vi "WriteResults - Rx.vi"(8 "error in (no error)":errorcluster, 9 "PSR":dbl, 11 "refnum out":refnum<file>) -> (0 "error out":errorcluster, 3 "refnum out 2":refnum<file>)   [LabVIEW 2012]
panel:
  out "concatenated string":string
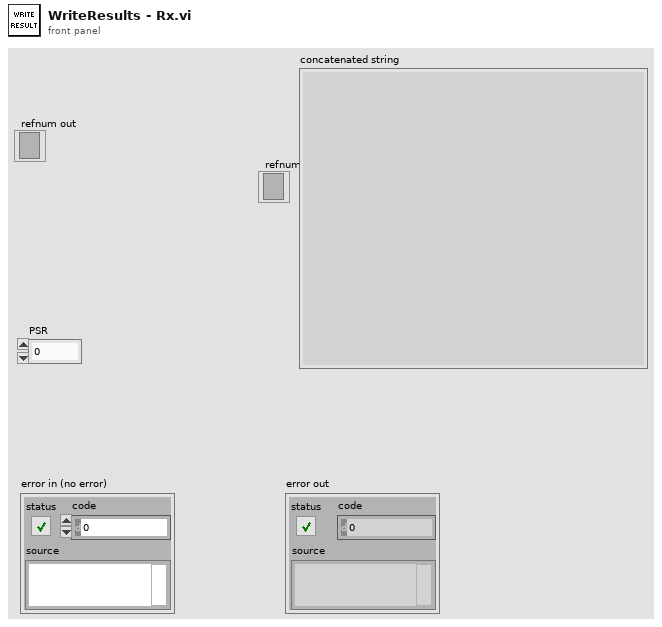
[diagram p1: front panel]
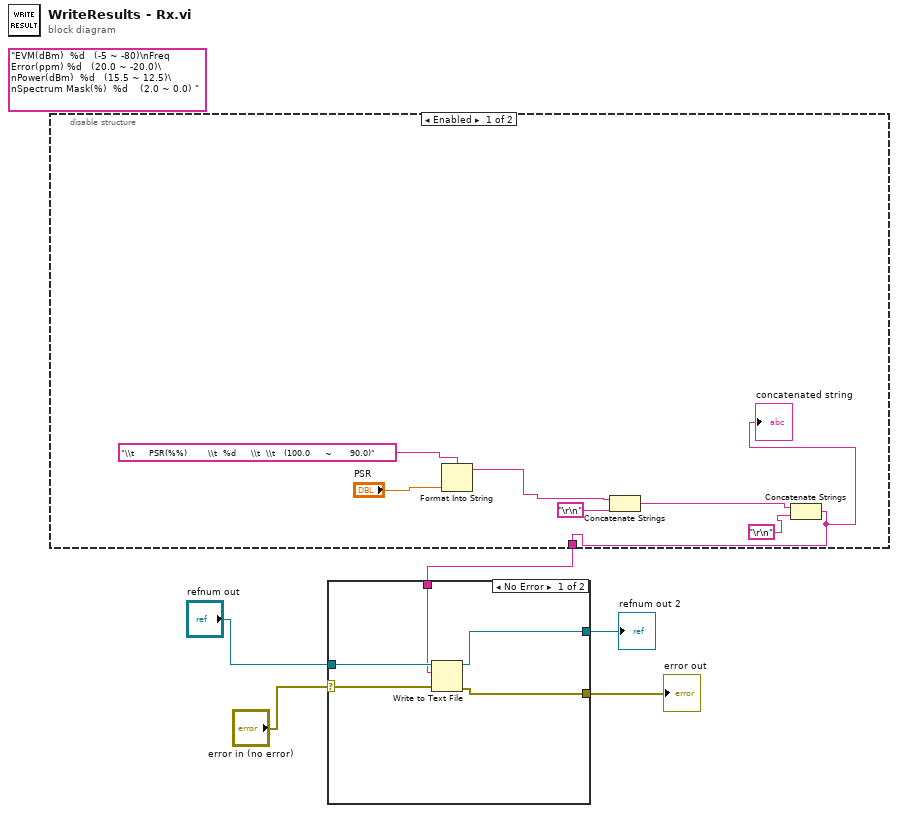
[diagram p0: block diagram]
diagram:
  (unwired) "EVM(dBm)  %d   (-5 ~ -80)\nFreq Error(ppm) %d   (20.0 ~ -20.0)\nPower(dBm)  %d   (15.5 ~ 12.5)\nSpectrum Mask(%)  %d    (2.0 ~ 0.0) " ("format string")
  n1 = disable-structure shown="Enabled" {
    disable-tunnel: [w6 _] -> w2
    frame Enabled {
      n2 = Format Into String(format string="\\t     PSR(%%)       \\t  %d     \\t  \\t   (100.0     ~      90.0)" ("initial string"), "PSR") -> (resulting string=w9:string)  [unwired: 2 in, 1 out]
      n3 = Concatenate Strings(w9, "\r\n") -> (w7:string)
      n4 = Concatenate Strings(w7, "\r\n") -> (w6:string)
      "concatenated string" <- w6
    }
    frame Disabled {
    }
  }
  n5 = case shown="No Error" "error in (no error)" {
    selector: "error in (no error)" -> [w16 w18]
    tunnel: [w15 w18] -> w4
    tunnel: "refnum out" -> [w17 _]
    tunnel: w2 -> [w14 _]
    tunnel: [w13 _] -> w1
    frame No Error {
      n6 = Write to Text File(file (use dialog)=w17, text=w14, error in=w16) -> (refnum out=w13:refnum<file>, error out=w15:errorcluster)  [unwired: 1 in, 1 out]
    }
    frame Error {
    }
  }
  "error out" <- w4
  "refnum out 2" <- w1
